vi "update_dds_hardware.vi"(10 "DDS Update List":T2[](array[typedef]), 11 "DDS Devices":T1(array[cluster])=[{"PB Trigger Line"=4, "Sweeps"=FALSE, "Channel Name"="DDS Chan 1", "Device Description"="DDS1", "PB trig / Sequence"=TRUE, "Amp Lock"=FALSE, "SetList Display"=[TRUE, FALSE, FALSE]}]) -> (2 "Bytes Written":u32[](array[numeric]), 3 "Output Stings to DDS(s)":string[](array[string]))   [LabVIEW 2010]
uses:
  Controls/DDSUpdate.ctt
panel:
  # "Freq    Amp   Phase"
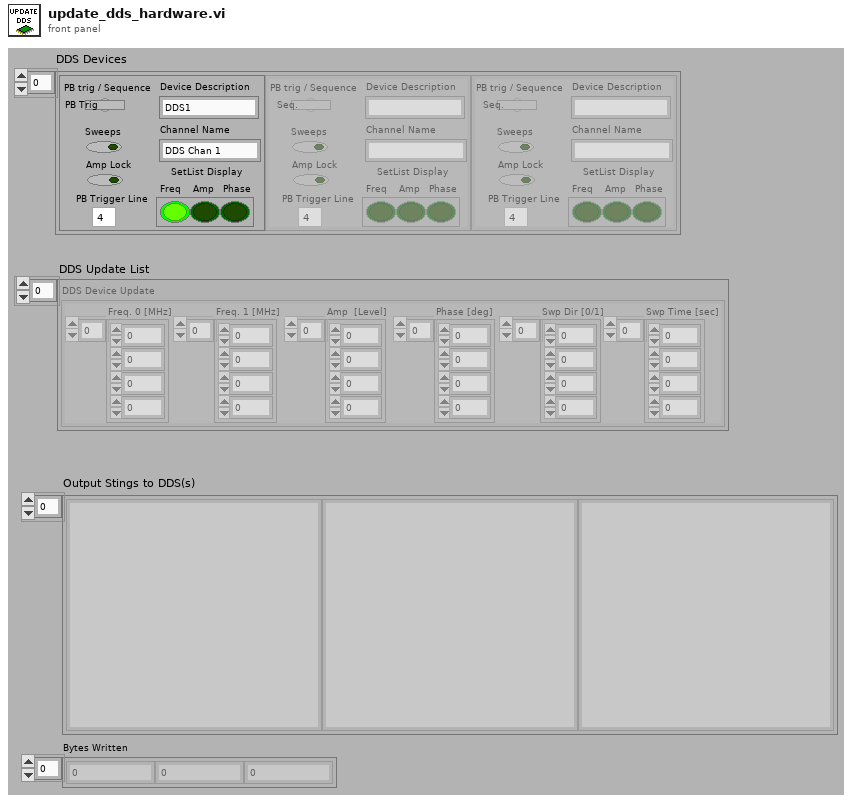
[diagram p1: front panel]
types:
  T1 = cluster{"PB Trigger Line":u16, "Sweeps":bool, "Channel Name":string, "Device Description":string, "PB trig / Sequence":bool, "Amp Lock":bool, "SetList Display":bool[]}[]
  T2 = typedef "DDSUpdate.ctt" = cluster{"Freq. 0 [MHz]":dbl[], "Amp  [Level]":dbl[], "Phase [deg]":dbl[], "Freq. 1 [MHz]":dbl[], "Swp Dir [0/1]":u16[], "Swp Time [sec]":dbl[]}
  T3 = cluster{"Freq. 0 [MHz]":dbl[], "Freq. 1 [MHz]":dbl[], "Amp  [Level]":dbl[], "Phase [deg]":dbl[], dbl[], "Swp Dir [0/1]":u16[], "Sweeps":bool, "Amp Lock":bool, bool}
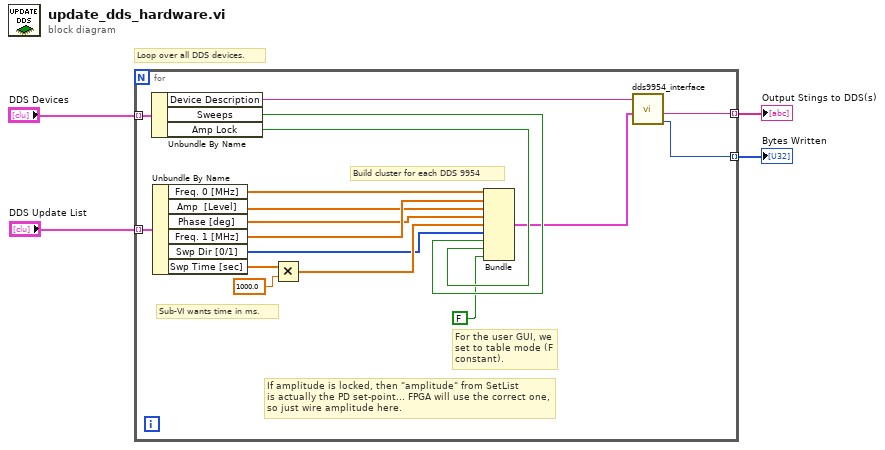
[diagram p0: block diagram]
diagram:
  # "Loop over all DDS devices."
  n1 = for {
    tunnel: "DDS Update List" -> [w21] mode=indexing
    tunnel: "DDS Devices" -> [w20] mode=indexing
    tunnel: [w18] -> w2 mode=indexing
    tunnel: [w17] -> w1 mode=indexing
    # "Sub-VI wants time in ms."
    # "Build cluster for each DDS 9954"
    # "For the user GUI, we\nset to table mode (F \nconstant)."
    # "If amplitude is locked, then \"amplitude\" from SetList\nis actually the PD set-point... FPGA will use the correct one,\nso just wire amplitude here."
    n2 = Unbundle By Name(w20) -> ("Device Description"=w19:string, "Sweeps"=w8:bool, "Amp Lock"=w7:bool)
    n3 = Unbundle By Name(w21) -> ("Freq. 0 [MHz]"=w16:dbl[], "Amp  [Level]"=w12:dbl[], "Phase [deg]"=w11:dbl[], "Freq. 1 [MHz]"=w13:dbl[], "Swp Dir [0/1]"=w9:u16[], "Swp Time [sec]"=w14:dbl[])
    n4 = Multiply(x=w14, y=1000.0) -> (x*y=w10:dbl[])
    n5 = Bundle("Freq. 0 [MHz]"=w16, "Freq. 1 [MHz]"=w13, "Amp  [Level]"=w12, "Phase [deg]"=w11, w10, "Swp Dir [0/1]"=w9, "Sweeps"=w8, "Amp Lock"=w7, FALSE) -> (w5:T3)  [unwired: 1 in]
    n6 = call "dds9954_interface.vi"("DDS 9954 Interface"=w5, "Device Description"=w19) -> ("Bytes Written"=w17:u32, "Characters to FPGA"=w18:string)  [unwired: 8 in]
  }
  "Output Stings to DDS(s)" <- w2
  "Bytes Written" <- w1
